vi "TurnLogic.vi"(9 "Goal Reached":bool=TRUE, 10 "Beta":dbl format="%#_13g", 11 "Delta Theta":dbl format="%#_13g") -> (3 "Increment Lean":i8)   [LabVIEW 2016]
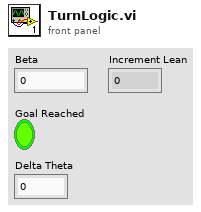
[diagram p1: front panel]
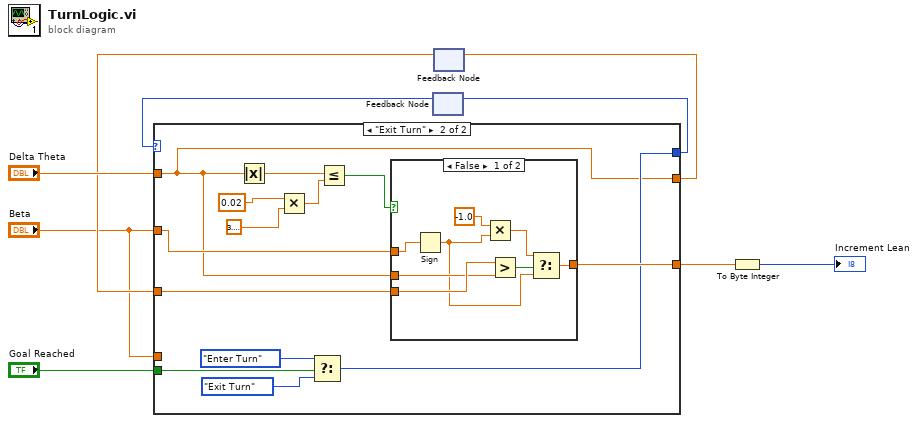
[diagram p0: block diagram]
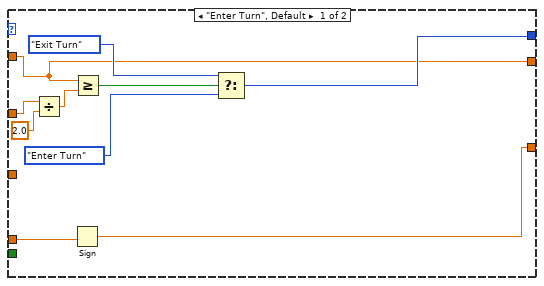
[diagram p2: hidden frame]
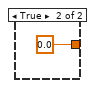
[diagram p3: hidden frame]
diagram:
  n1 = feedback #1() -> (w8:enum16{"Enter Turn", "Exit Turn"})  [unwired: 1 in]
  n2 = feedback #2() -> (w5:dbl)  [unwired: 1 in]
  n3 = case shown="\"Exit Turn\"" w8 {
    tunnel: [w13 w21] -> w9
    tunnel: "Beta" -> [w19 w25]
    tunnel: "Delta Theta" -> [w12 w20]
    tunnel: [w12 w20] -> w6
    tunnel: w5 -> [_ w26]
    tunnel: [w10 w27] -> w1
    tunnel: "Beta" -> [w11 _]
    tunnel: "Goal Reached" -> [_ w24]
    frame "Enter Turn", Default {
      n4 = Divide(x=w19, y=2.0) -> (x/y=w17:dbl)
      n5 = Sign(1:w11) -> (0:w10:dbl)
      n6 = Greater Or Equal?(x=w12, y=w17) -> (x >= y?=w16:bool)
      n7 = Select(t=enum16{"Enter Turn", "Exit Turn"}."Exit Turn", s=w16, f=enum16{"Enter Turn", "Exit Turn"}."Enter Turn") -> (s? t:f=w13:enum16{"Enter Turn", "Exit Turn"})
    }
    frame "Exit Turn" {
      n8 = Absolute Value(x=w20) -> (abs(x)=w32:dbl)
      n9 = Multiply(x=0.02, y=3.141592653589793) -> (x*y=w29:dbl)
      n10 = Select(t=enum16{"Enter Turn", "Exit Turn"}."Enter Turn", s=w24, f=enum16{"Enter Turn", "Exit Turn"}."Exit Turn") -> (s? t:f=w21:enum16{"Enter Turn", "Exit Turn"})
      n11 = Less Or Equal?(x=w32, y=w29) -> (x <= y?=w28:bool)
      n12 = case shown="False" w28 {
        tunnel: [w34 0.0] -> w27
        tunnel: w26 -> [w40 _]
        tunnel: w20 -> [w39 _]
        tunnel: w25 -> [w35 _]
        frame False {
          n13 = Sign(1:w35) -> (0:w33:dbl)
          n14 = Multiply(x=-1.0, y=w33) -> (x*y=w36:dbl)
          n15 = Greater?(x=w40, y=w39) -> (0:w38:bool)
          n16 = Select(t=w36, s=w38, f=w33) -> (s? t:f=w34:dbl)
        }
        frame True {
        }
      }
    }
  }
  n17 = feedback-in #1(w9) -> ()
  n18 = feedback-in #2(w6) -> ()
  n19 = To Byte Integer(number=w1) -> (8bit integer=→"Increment Lean":i8)
